vi "Read Control Limits.vi"(8 "error in":errorcluster, 11 "Has Control Limits in":refnum<class "Has Control Limits.lvclass">) -> (0 "error out":errorcluster, 2 "control limits":T1, 3 "Has Control Limits out":refnum<class "Has Control Limits.lvclass">)   [LabVIEW 2020, in "PV Access.lvlib" / "PV Data.lvlib" / "Has Control Limits.lvclass"]
uses:
  Has Control Limits.lvclass
  182da66a-f6ee-47d3-9b05-9cecdf4c7a27.vi
  Control Metadata.ctl
  PV Data.lvlib
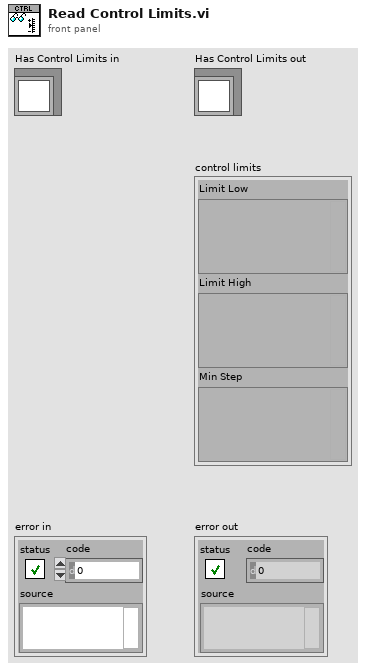
[diagram p1: front panel]
types:
  T1 = typedef "PV Access.lvlib/PV Data.lvlib/Control Metadata.ctl" = cluster{"Limit Low":variant, "Limit High":variant, "Min Step":variant}
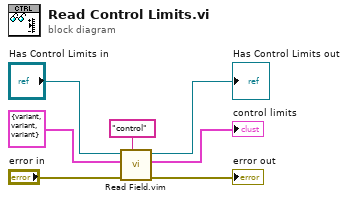
[diagram p0: block diagram]
diagram:
  n1 = call "Read Field.vim"("field"="control" ("element name"), "error in"="error in", "default value"=T1 {"Limit Low"=variant, "Limit High"=variant, "Min Step"=variant} ("Control Metadata"), "Base Interface in"="Has Control Limits in") -> ("error out"=→"error out":errorcluster, "value"=→"control limits":T1, "Base Interface out"=→"Has Control Limits out":refnum<class "Has Control Limits.lvclass">)  [unwired: 5 in]
